vi "PhotonTargetModel_New.vi"(9 "IsSpherical":bool, 10 "IsPlaner":bool, 11 "Vertices":T1[](array[typedef]) {"Z" format="%14.3f"; "Y" format="%14.3f"; "X" format="%14.3f"}) -> (3 "PhotonTargetModel":T2 {"Vertices"."Z" format="%14.3f"; "Vertices"."Y" format="%14.3f"; "Vertices"."X" format="%14.3f"})   [LabVIEW 2019, in "PhotonVisionLib.lvlib"]
doc: "Creates a rectangular, planar target model given the verticies and type information.. \n\nInputs:\n - veerticies -- Translation3d array - \n - IsPlanar - boolean\n - IsSpherical - boolean\n\nOutputs:\n - TargetModel - cluster - created target model"
uses:
  PhotonVisionLib.lvlib
  TypeDef/PhotonTargetModel.ctl
  <vilib>/Rock Robotics/WPI/ThirdParty/JAS_Junk/TrajLib/TypeDef/TRANSLATION3D.ctl
  <vilib>/Rock Robotics/WPI/ThirdParty/JAS_Junk/TrajLib/Trajectory_Library.lvlib
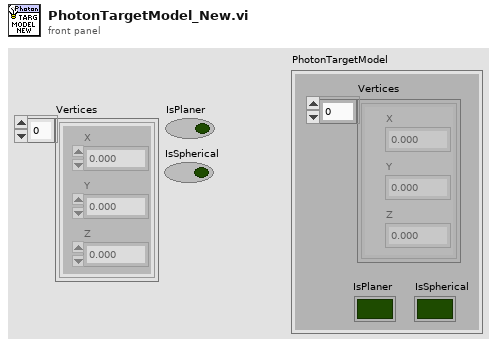
[diagram p1: front panel]
types:
  T1 = typedef "Trajectory_Library.lvlib/TRANSLATION3D.ctl" = cluster{"X":dbl, "Y":dbl, "Z":dbl}
  T2 = typedef "PhotonVisionLib.lvlib/PhotonTargetModel.ctl" = cluster{"Vertices":T1[], "IsPlaner":bool, "IsSpherical":bool}
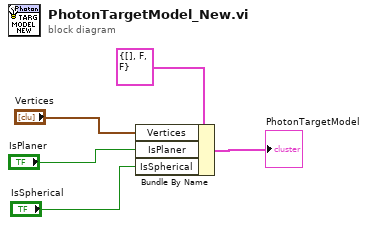
[diagram p0: block diagram]
diagram:
  n1 = Bundle By Name(cluster=T2 {"Vertices"=[], "IsPlaner"=FALSE, "IsSpherical"=FALSE} ("PhotonTargetModel"), "Vertices"="Vertices", "IsPlaner"="IsPlaner", "IsSpherical"="IsSpherical") -> (→"PhotonTargetModel":T2)
